vi "Data_Save.vi"(7 "AllControls In":T2, 8 "Data in":T1) -> ()   [LabVIEW 2017]
uses:
  Ctrls/AllControls.ctl
  Ctrls/CSV_Data.ctl
  <vilib>/Utility/file.llb/Write Delimited Spreadsheet (string).vi
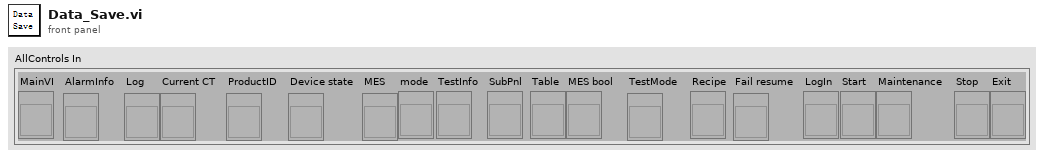
[diagram p1: front panel]
types:
  T1 = typedef "CSV_Data.ctl" = cluster{"Version":cluster{"SC_Version":string, "VP_Version":string}, "SN":string, "Table":string[][], "Count":cluster{"Total":i32, "OK":i32, "NG":i32, "Yield":dbl}, "Start Time":timestamp, "daemon reference":refnum<k5>, "CT":dbl, "Config":string[][], "OK/NG":bool, "Station ID":string, "MES DDM SN":string, "MES PCBA SN":string, "Retest":string, "Lux":string, "VOT":cluster{"Initial brightness":string, "Mean uniformity":string, "Uniformity_Deviation":string, "Adjusted brightness":string, "Mean_Adjusted":string, "Deviation_Adjusted":string, "Reflection":string, "Result":bool}, "SKU":string, "Plate_Diameter":string, "Alarm":string}
  T2 = typedef "AllControls.ctl" = cluster{"MainVI":refnum<vi>, "AlarmInfo":refnum<vi>, "Log":refnum<vi>, "Current CT":refnum<vi>, "ProductID":refnum<vi>, "Device state":refnum<vi>, "MES":refnum<vi>, "mode":refnum<vi>, "TestInfo":refnum<vi>, "SubPnl":refnum<vi>, "Table":refnum<vi>, "MES bool":refnum<vi>, "TestMode":refnum<vi>, "Recipe":refnum<vi>, "Fail resume":refnum<vi>, "LogIn":refnum<vi>, "Start":refnum<vi>, "Maintenance":refnum<vi>, "Stop":refnum<vi>, "Exit":refnum<vi>}
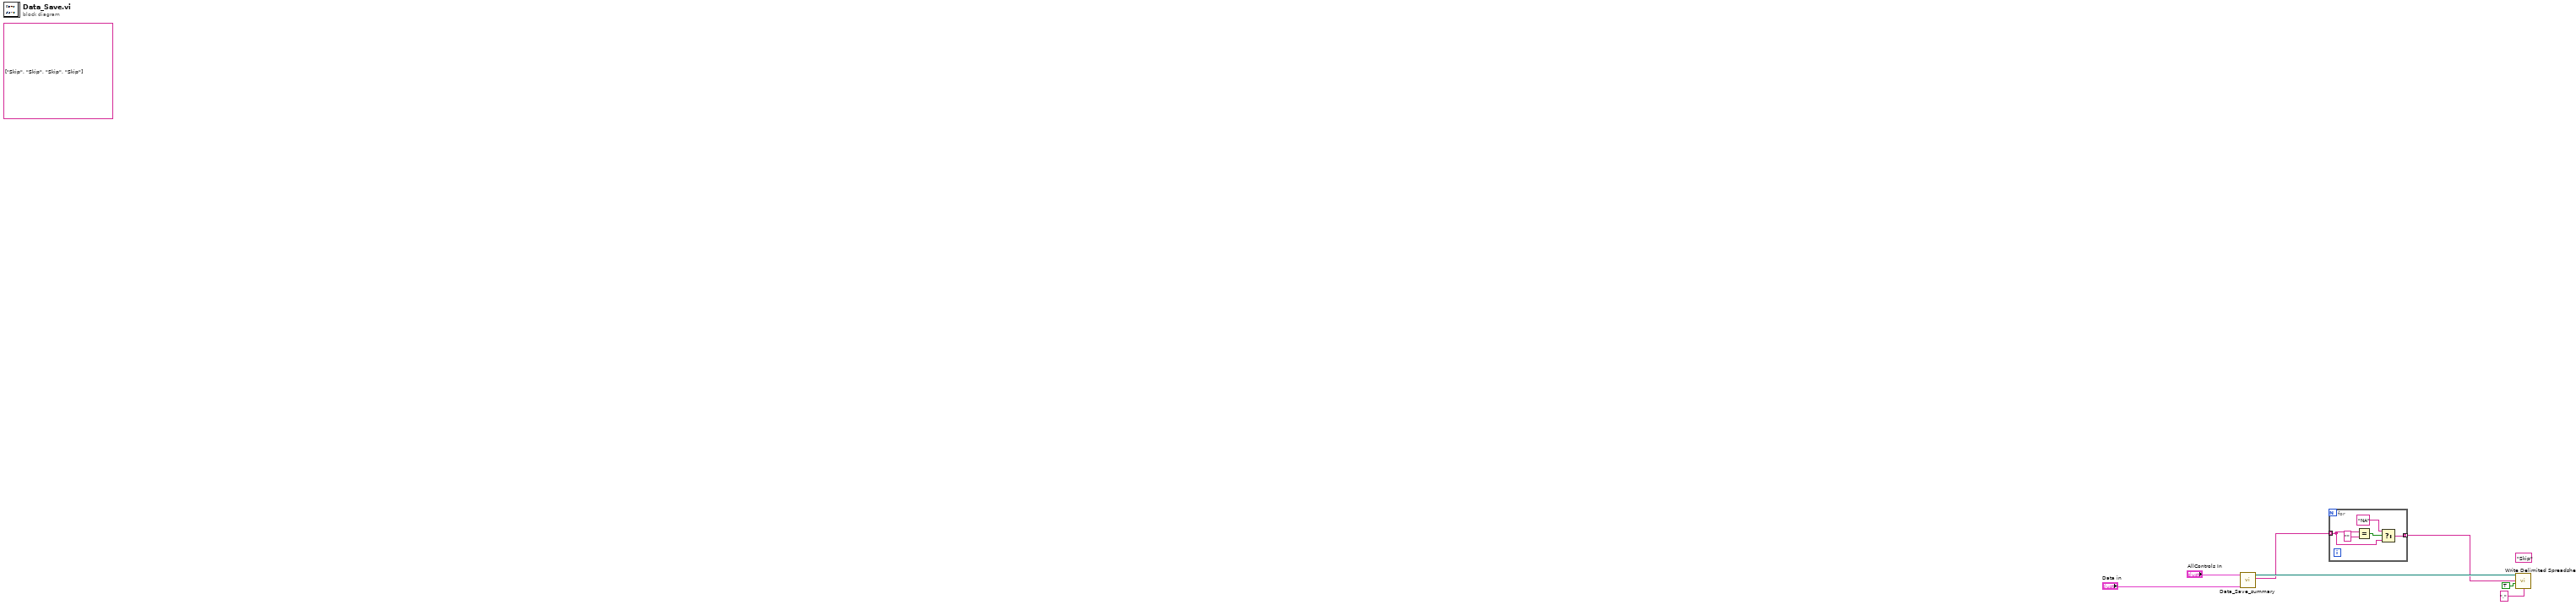
[diagram p0: block diagram]
diagram:
  (unwired) string[] ["Skip", "Skip", "Skip", "Skip"]
  (unwired) "Skip" ("x")
  n1 = call "Data_Save_summary.vi"("Data in"="Data in", "AllControls In"="AllControls In") -> ("data"=w1:string[], "dup path"=w5:path)  [unwired: 8 in]
  n2 = for {
    tunnel: w1 -> [w9] mode=indexing
    tunnel: [w8] -> w2 mode=indexing
    n3 = Equal?(x=w9, y="") -> (x = y?=w11:bool)
    n4 = Select(t="NA" ("y"), s=w11, f=w9) -> (s? t:f=w8:string)
  }
  n5 = call-poly <vilib>:"Write Delimited Spreadsheet.vi"("file path (dialog if empty)"=w5, "1D data"=w2, "append to file? (new file:F)"=TRUE, "delimiter (\\t)"="," ("delimiter (\\t)")) -> ()  [unwired: 10 in, 2 out]
